vi "Setra Read Write.vi"(8 "Error In":errorcluster, 10 "Setra Command":T1="#", 11 "VISA (Input)":refnum<visa-resource-name>) -> (0 "Error Out":errorcluster, 2 "read buffer":string, 3 "VISA Refnum (Output)":refnum<visa-resource-name>)   [LabVIEW 2016]
uses:
  Type Definitions/Setra Commands.ctl
panel:
  out "Serial Settings:Number of Bytes at Serial Port":u32
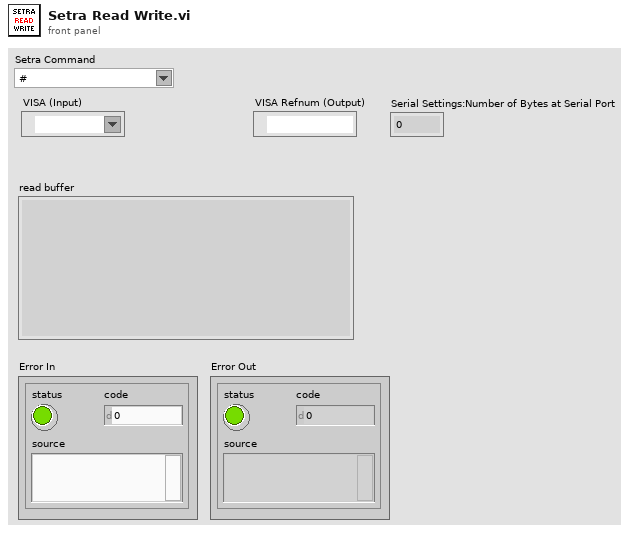
[diagram p1: front panel]
types:
  T1 = typedef "Setra Commands.ctl" = string
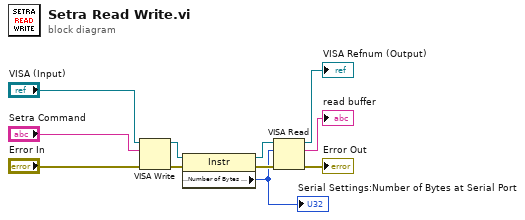
[diagram p0: block diagram]
diagram:
  n1 = VISA Write(VISA resource name="VISA (Input)", write buffer="Setra Command", error in (no error)="Error In") -> (VISA resource name out=w8:refnum<visa-resource-name>, error out=w7:errorcluster)  [unwired: 1 out]
  n2 = property class="Instr"(reference=w8, error in=w7) -> (reference out=w5:refnum<visa-resource-name>, error out=w6:errorcluster, "Serial Settings:Number of Bytes at Serial Port"=w4:u32)
  "Serial Settings:Number of Bytes at Serial Port" <- w4
  n3 = VISA Read(VISA resource name=w5, byte count=w4, error in (no error)=w6) -> (VISA resource name out=→"VISA Refnum (Output)":refnum<visa-resource-name>, read buffer=→"read buffer":string, error out=→"Error Out":errorcluster)  [unwired: 1 out]
